vi "readws.vi"(11 "Path":path) -> (0 "error out":errorcluster, 3 "Array":T1[](array[typedef]))   [LabVIEW 2013]
uses:
  ws.ctl
  <resource>/Framework/Providers/ws_project_provider/common/Web Service.ctl
  <resource>/Framework/Providers/ws_project_provider/common/Web Service VI.ctl
  <resource>/Framework/Providers/ws_project_provider/common/Web Service VI Type.ctl
  <resource>/Framework/Providers/ws_project_provider/common/Web Service VI Method.ctl
  <resource>/Framework/Providers/ws_project_provider/common/Web Service VI Output Type.ctl
  <resource>/Framework/Providers/ws_project_provider/common/Web Service VI Output Format.ctl
  <resource>/Framework/Providers/ws_project_provider/common/NI Web Service Provider.lvlib
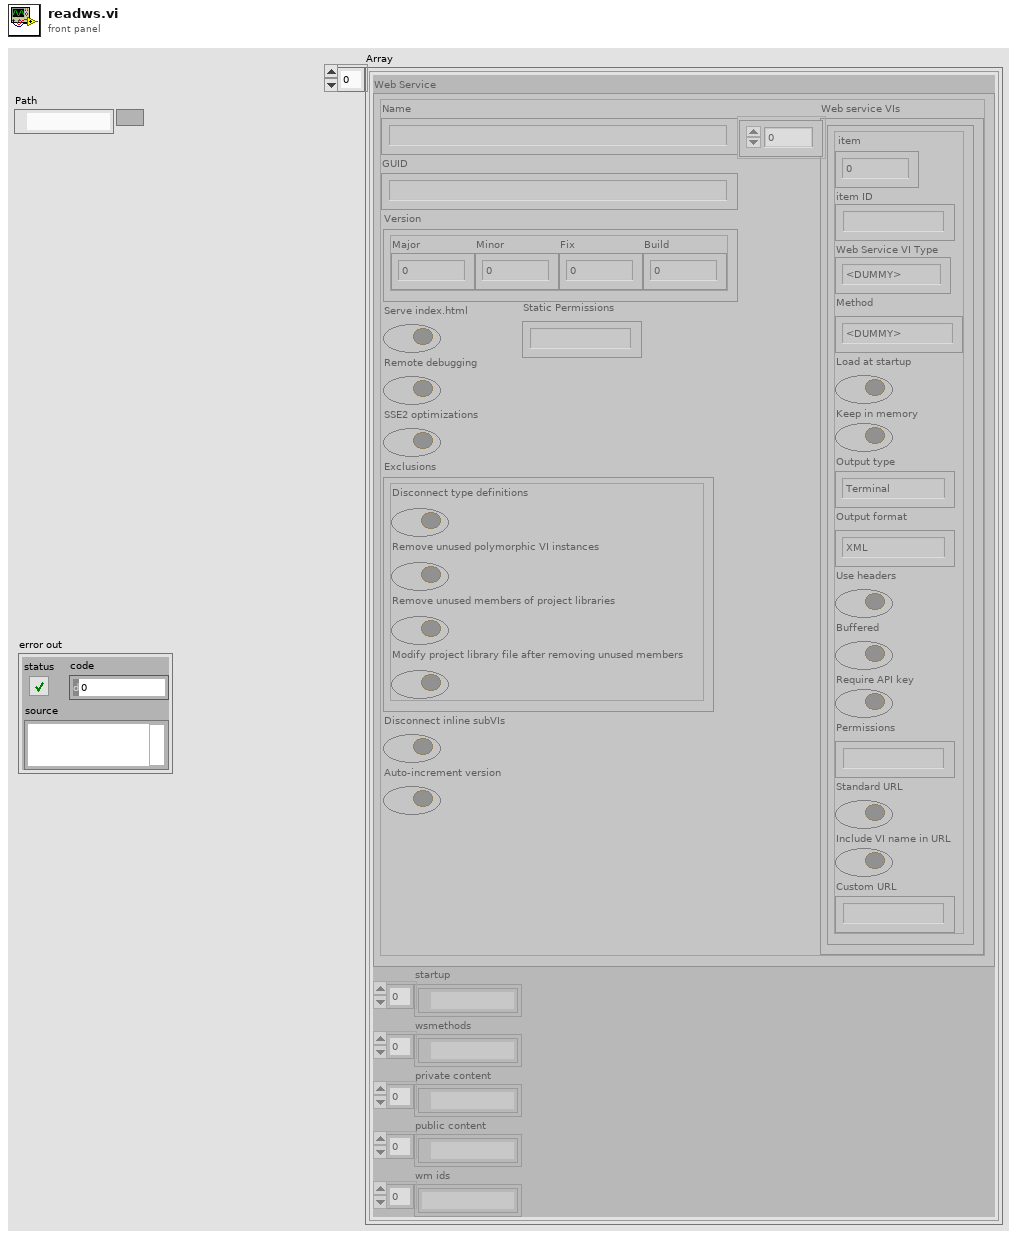
[diagram p1: front panel]
types:
  T1 = typedef "ws.ctl" = cluster{"Web Service":T2, "startup":path[], "wsmethods":path[], "private content":path[], "public content":path[], "wm ids":string[]}
  T2 = typedef "NI Web Service Provider.lvlib/Web Service.ctl" = cluster{"Name":string, "GUID":string, "Version":cluster{"Major":u16, "Minor":u16, "Fix":u16, "Build":u16}, "Serve index.html":bool, "Remote debugging":bool, "SSE2 optimizations":bool, "Exclusions":cluster{"Disconnect type definitions":bool, "Remove unused polymorphic VI instances":bool, "Remove unused members of project libraries":bool, "Modify project library file after removing unused members":bool}, "Disconnect inline subVIs":bool, "Auto-increment version":bool, "Web service VIs":T3[], "Static Permissions":string}
  T3 = typedef "NI Web Service Provider.lvlib/Web Service VI.ctl" = cluster{"item":u64, "item ID":string, "Web Service VI Type":T4, "Method":T5, "Load at startup":bool, "Keep in memory":bool, "Output type":T6, "Output format":T7, "Use headers":bool, "Buffered":bool, "Require API key":bool, "Permissions":string, "Standard URL":bool, "Include VI name in URL":bool, "Custom URL":string}
  T4 = typedef "NI Web Service Provider.lvlib/Web Service VI Type.ctl" = enum16{"<DUMMY>", "Web Method", "Auxiliary", "Internal", "Content"}
  T5 = typedef "NI Web Service Provider.lvlib/Web Service VI Method.ctl" = enum16{"<DUMMY>", "GET", "PUT", "POST", "DELETE", "OPTIONS", "HEAD", "TRACE"}
  T6 = typedef "NI Web Service Provider.lvlib/Web Service VI Output Type.ctl" = enum16{"Terminal", "Stream"}
  T7 = typedef "NI Web Service Provider.lvlib/Web Service VI Output Format.ctl" = enum16{"<DUMMY>", "Text", "XML", "HTML", "JSON"}
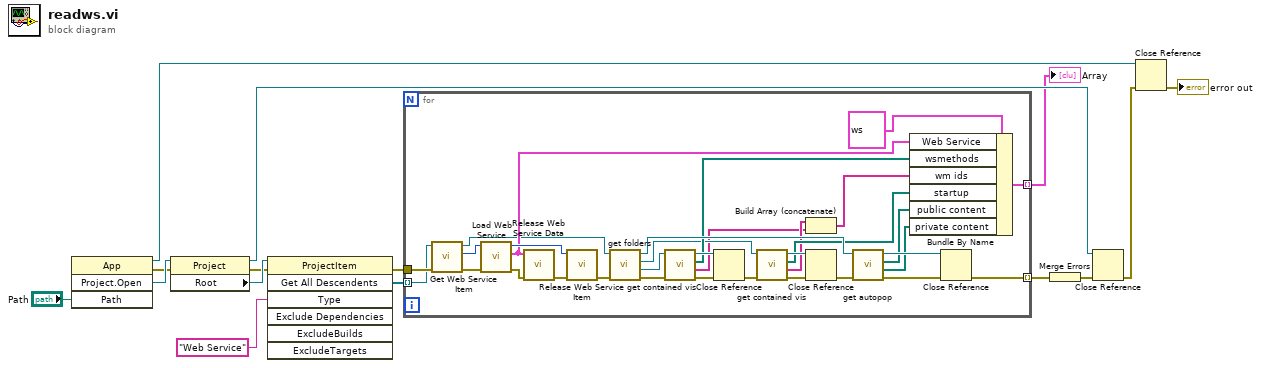
[diagram p0: block diagram]
diagram:
  n1 = invoke class="App" method="Project.Open"("Path"="Path") -> (reference out=w15:refnum<vi>, error out=w4:errorcluster, "Project:Open"=w12:refnum<vi>)  [unwired: 3 in, 1 out]
  n2 = property class="Project"(reference=w12, error in=w4) -> (reference out=w13:refnum<vi>, error out=w5:errorcluster, "Root"=w11:refnum<vi>)
  n3 = invoke class="ProjectItem" method="Get All Descendents"(reference=w11, error in=w5, "Type"="Web Service") -> (error out=w6:errorcluster, "All Descendents"=w10:refnum<vi>[])  [unwired: 4 in, 5 out]
  n4 = for {
    tunnel: w10 -> [w40] mode=indexing
    tunnel: [w41] -> w8 mode=indexing
    tunnel: w6 -> [w43]
    tunnel: [w35] -> w2 mode=indexing
    n5 = call <resource>:"Get Web Service Item.vi"("Error In"=w43, "Web service project item"=w40) -> ("Error Out"=w46:errorcluster, "Web service item"=w47:u64, "Web service project item out"=w34:refnum<vi>)  [unwired: 7 in]
    n6 = call <resource>:"Load Web Service.vi"("Error In"=w46, "Web service item"=w47) -> ("Error Out"=w44:errorcluster, "Web Service"=w36:T2, "Web service item out"=w42:u64)  [unwired: 7 in]
    n7 = call <resource>:"Release Web Service Data.vi"("Error In"=w44, "Web Service"=w36) -> ("Error Out"=w45:errorcluster)  [unwired: 9 in]
    n8 = call <resource>:"Release Web Service Item.vi"("Error In"=w45, "Web service item"=w42) -> ("Error Out"=w33:errorcluster)  [unwired: 9 in]
    n9 = call "get folders.vi"("error in"=w33, "web service in"=w34) -> ("error out"=w21:errorcluster, "web methods"=w23:refnum<vi>, "startup"=w22:refnum<vi>, "Web service project item out"=w30:refnum<vi>)  [unwired: 6 in]
    n10 = call "get contained vis.vi"("error in"=w21, "ProjectItem in"=w23) -> ("error out"=w32:errorcluster, "ids"=w17:string[], "paths"=w24:path[], "ProjectItem out"=w31:refnum<vi>)  [unwired: 6 in]
    n11 = Close Reference(reference=w31, error in (no error)=w32) -> (error out=w26:errorcluster)
    n12 = call "get contained vis.vi"("error in"=w26, "ProjectItem in"=w22) -> ("error out"=w29:errorcluster, "ids"=w18:string[], "paths"=w25:path[], "ProjectItem out"=w27:refnum<vi>)  [unwired: 6 in]
    n13 = Build Array (concatenate)(w18, w17) -> (w16:string[])
    n14 = Close Reference(reference=w27, error in (no error)=w29) -> (error out=w28:errorcluster)
    n15 = call "get autopop.vi"("error in"=w28, "ProjectItem in"=w30) -> ("error out"=w38:errorcluster, "private"=w20:path[], "public"=w19:path[], "ProjectItem out"=w39:refnum<vi>)  [unwired: 6 in]
    n16 = Bundle By Name(cluster=T1 {"Web Service"={"Name"="", "GUID"="", "Version"={"Major"=0, "Minor"=0, "Fix"=0, "Build"=0}, "Serve index.html"=FALSE, "Remote debugging"=FALSE, "SSE2 optimizations"=FALSE, "Exclusions"={"Disconnect type definitions"=FALSE, "Remove unused polymorphic VI instances"=FALSE, "Remove unused members of project libraries"=FALSE, "Modify project library file after removing unused members"=FALSE}, "Disconnect inline subVIs"=FALSE, "Auto-increment version"=FALSE, "Web service VIs"=[], "Static Permissions"=""}, "startup"=[], "wsmethods"=[], "private content"=[], "public content"=[], "wm ids"=[]} ("ws"), "Web Service"=w36, "wsmethods"=w24, "wm ids"=w16, "startup"=w25, "public content"=w19, "private content"=w20) -> (w35:T1)
    n17 = Close Reference(reference=w39, error in (no error)=w38) -> (error out=w41:errorcluster)
  }
  "Array" <- w2
  n18 = Merge Errors(w8) -> (w7:errorcluster)
  n19 = Close Reference(reference=w13, error in (no error)=w7) -> (error out=w14:errorcluster)
  n20 = Close Reference(reference=w15, error in (no error)=w14) -> (error out=→"error out":errorcluster)
